vi "GetProtocolSection.vi"(8 "error in (no error)":errorcluster caption="에러 입력(에러 없음)", 10 "SectionMap":T1, 11 "ABFFIO 입력":refnum<class "ABFFIO.lvclass">) -> (0 "error out":errorcluster caption="에러 출력", 3 "ABFFIO 출력":refnum<class "ABFFIO.lvclass">)   [LabVIEW 2017, in "ABFFIO.lvclass"]
uses:
  ABFFIO.lvclass
  ABFFIO.lvclass/ABFFIO.ctl
panel:
  out "SecPerPoint":dbl
  out "Samplingrate":i32
  out "MumSamplesPerEpisode":u32
  out "OperationMode":u8
  out "DACRange":sgl
  out "ADCRange":sgl
  out "ADCSequenceInterval":sgl
  out "DACResolution":u32
  out "ADCResolution":u32
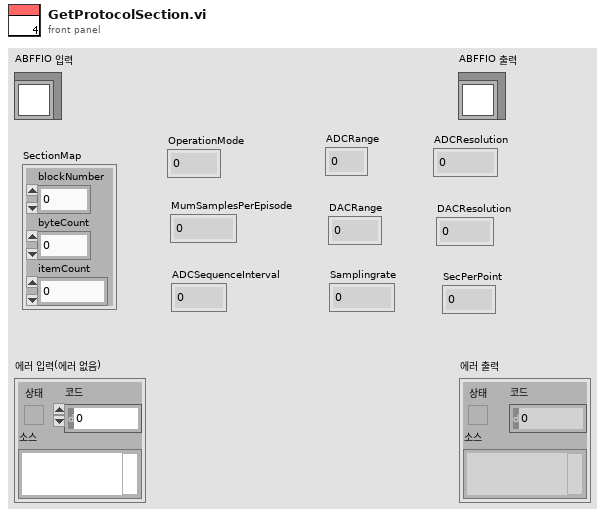
[diagram p1: front panel]
types:
  T1 = cluster{"blockNumber":u32, "byteCount":u32, "itemCount":u32}
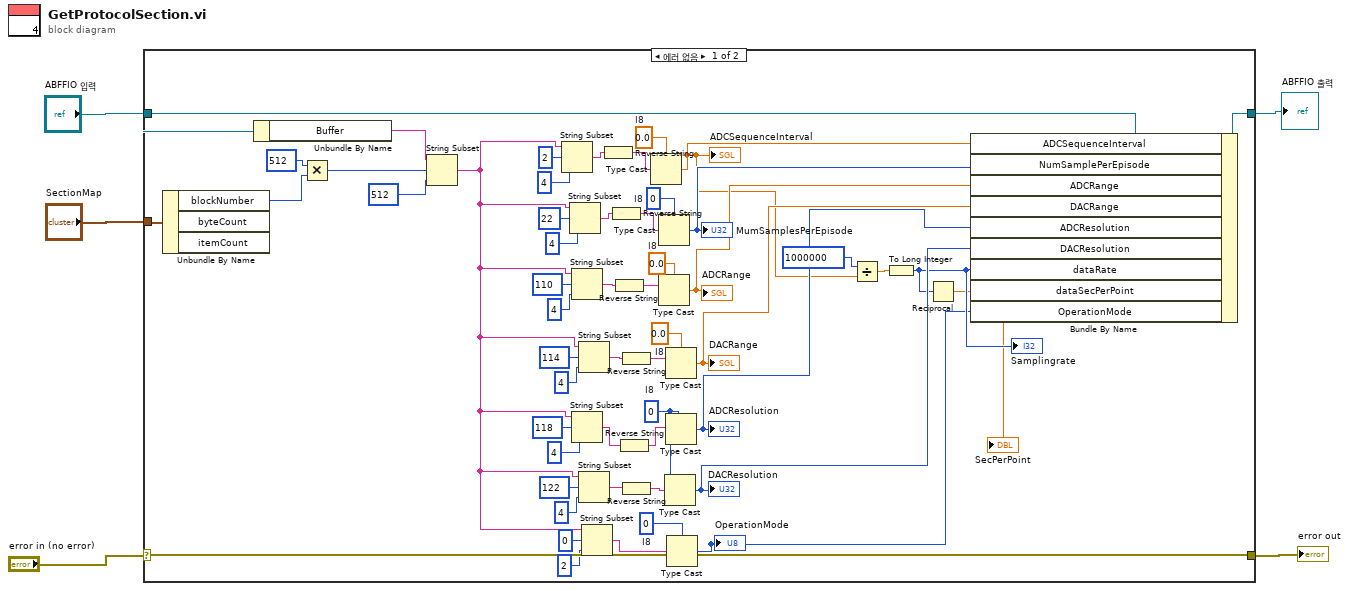
[diagram p0: block diagram]
diagram:
  n1 = case shown="에러 없음" "error in (no error)" {
    selector: "error in (no error)" -> [w59 w61]
    tunnel: [w59 w61] -> w4
    tunnel: [w24 w60] -> w2
    tunnel: "ABFFIO 입력" -> [w29 w60]
    tunnel: "SectionMap" -> [w35 _]
    frame No Error {
      w18 = u32 0  # I8
      w20 = u8 0  # I8
      w30 = sgl 0.0  # I8
      w37 = sgl 0.0  # I8
      w38 = sgl 0.0  # I8
      w39 = u32 0  # I8
      n2 = Unbundle By Name(w35) -> ("blockNumber"=w58:u32)  [unwired: 2 out]
      n3 = Unbundle By Name(w29) -> ("Buffer"=w55:string)
      n4 = Multiply(x=512, y=w58) -> (x*y=w56:u32)
      n5 = String Subset(string=w55, offset (0)=w56, length (rest)=i16 512) -> (substring=w13:string)
      n6 = String Subset(string=w13, offset (0)=i16 2 ("오프셋(0)"), length (rest)=4 ("길이(나머지)")) -> (substring=w41:string)
      n7 = String Subset(string=w13, offset (0)=i16 22 ("오프셋(0)"), length (rest)=4 ("길이(나머지)")) -> (substring=w16:string)
      n8 = String Subset(string=w13, offset (0)=110 ("오프셋(0)"), length (rest)=4 ("길이(나머지)")) -> (substring=w47:string)
      n9 = String Subset(string=w13, offset (0)=i16 118 ("오프셋(0)"), length (rest)=4 ("길이(나머지)")) -> (substring=w52:string)
      n10 = String Subset(string=w13, offset (0)=114 ("오프셋(0)"), length (rest)=4 ("길이(나머지)")) -> (substring=w31:string)
      n11 = String Subset(string=w13, offset (0)=i16 122 ("오프셋(0)"), length (rest)=4 ("길이(나머지)")) -> (substring=w21:string)
      n12 = String Subset(string=w13, offset (0)=i16 0 ("오프셋(0)"), length (rest)=2 ("길이(나머지)")) -> (substring=w19:string)
      n13 = Reverse String(1:w41) -> (0:w40:string)
      n14 = Reverse String(1:w16) -> (0:w17:string)
      n15 = Reverse String(1:w47) -> (0:w36:string)
      n16 = Reverse String(1:w52) -> (0:w51:string)
      n17 = Reverse String(1:w31) -> (0:w34:string)
      n18 = Reverse String(1:w21) -> (0:w42:string)
      n19 = Type Cast(type=w38, x=w40) -> (*(type *) &x=w10:sgl)
      "ADCSequenceInterval" <- w10
      n20 = Type Cast(type=w18, x=w17) -> (*(type *) &x=w12:u32)
      "MumSamplesPerEpisode" <- w12
      n21 = Type Cast(type=w37, x=w36) -> (*(type *) &x=w28:sgl)
      "ADCRange" <- w28
      n22 = Type Cast(type=w39, x=w42) -> (*(type *) &x=w25:u32)
      "DACResolution" <- w25
      n23 = Type Cast(type=w30, x=w34) -> (*(type *) &x=w27:sgl)
      "DACRange" <- w27
      n24 = Type Cast(type=w39, x=w51) -> (*(type *) &x=w26:u32)
      "ADCResolution" <- w26
      n25 = Type Cast(type=w20, x=w19) -> (*(type *) &x=w6:u8)
      "OperationMode" <- w6
      n26 = Divide(x=1000000, y=w10) -> (x/y=w9:sgl)
      n27 = To Long Integer(number=w9) -> (32bit integer=w8:i32)
      "Samplingrate" <- w8
      n28 = Reciprocal(x=w8) -> (1/x=w7:dbl)
      "SecPerPoint" <- w7
      n29 = Bundle By Name(cluster=w29, "ADCSequenceInterval"=w10, "NumSamplePerEpisode"=w12, "ADCRange"=w28, "DACRange"=w27, "ADCResolution"=w26, "DACResolution"=w25, "dataRate"=w8, "dataSecPerPoint"=w7, "OperationMode"=w6) -> (w24:refnum<class "ABFFIO.lvclass">)
    }
    frame Error {
    }
  }
  "error out" <- w4
  "ABFFIO 출력" <- w2
